vi "MinimalLiveExample.vi"() -> ()   [LabVIEW 2020]
uses:
  C:/Users/Public/Documents/Photometrics/TPM-LabVIEWSamples/Examples/2020/Dependencies/PVCamNET.dll
  Public/Documents/Photometrics/TPM-LabVIEWSamples/Examples/2020/Dependencies/PVCamNET.dll
panel:
  in  "Stop":bool
  out "Image Data":u16[][](array[numeric])
  out "Error":errorcluster
  out "Current Frame":u32
  out "Sensor Width":u32
  out "Sensor Height":u32
  out "Camera Name":string
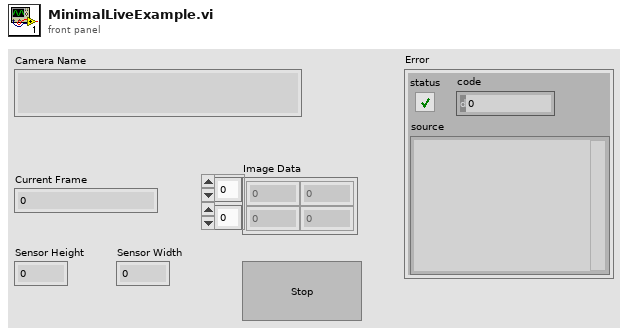
[diagram p1: front panel]
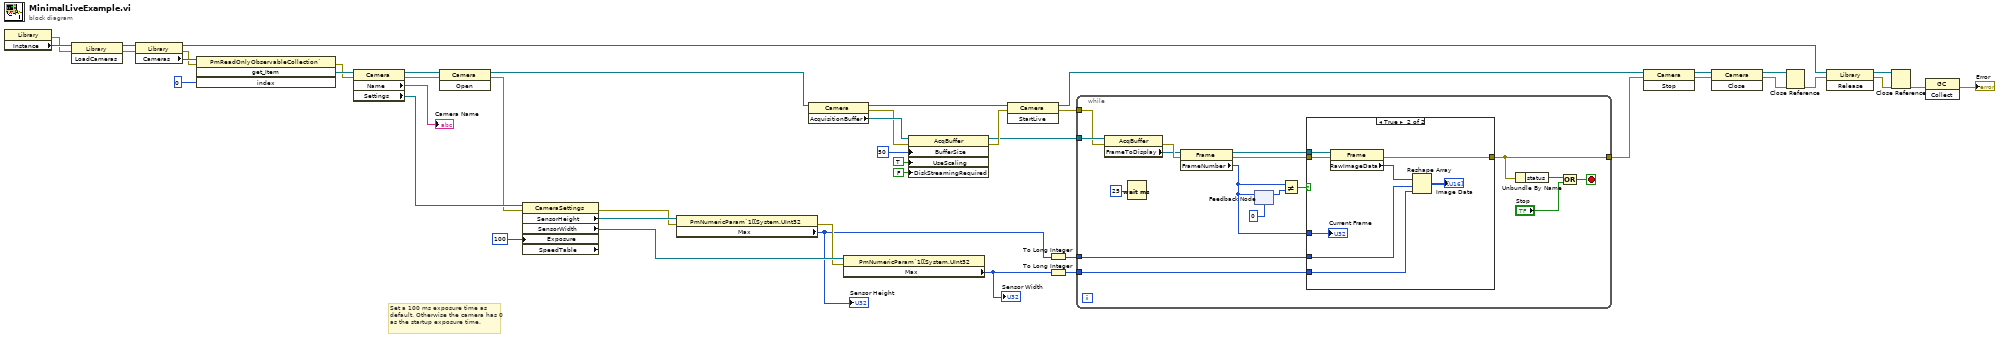
[diagram p0: block diagram]
diagram:
  # "Set a 100 ms exposure time as default. Otherwise the camera has 0 as the startup exposure time."
  n1 = property class="Library"() -> (error out=w42:errorcluster, "Instance"=w45:refnum<k24>)  [unwired: 2 in, 1 out]
  n2 = invoke class="Library" method="LoadCameras"(reference=w45, error in=w42) -> (reference out=w44:refnum<k24>, error out=w41:errorcluster)  [unwired: 1 in, 1 out]
  n3 = property class="Library"(reference=w44, error in=w41) -> (reference out=w34:refnum<k24>, error out=w40:errorcluster, "Cameras"=w43:refnum<k24>)
  n4 = invoke class="PmReadOnlyObservableCollection`" method="get_Item"(reference=w43, error in=w40, "index"=0) -> (error out=w38:errorcluster, "get_Item"=w39:refnum<k24>)  [unwired: 1 in, 2 out]
  n5 = property class="Camera"(reference=w39, error in=w38) -> (reference out=w36:refnum<k24>, error out=w33:errorcluster, "Name"=→"Camera Name":string, "Settings"=w37:refnum<k24>)
  n6 = invoke class="Camera" method="Open"(reference=w36, error in=w33) -> (reference out=w7:refnum<k24>, error out=w32:errorcluster)  [unwired: 1 in, 1 out]
  n7 = property class="CameraSettings" props=["SensorHeight", "SensorWidth", "Exposure", "SpeedTable"](reference=w37, error in=w32, "Exposure"=u32 100) -> (error out=w29:errorcluster, "SensorHeight"=w31:refnum<k24>, "SensorWidth"=w30:refnum<k24>)  [unwired: 2 out]
  n8 = property class="PmNumericParam`1[[System.UInt32"(reference=w31, error in=w29) -> (error out=w28:errorcluster, "Max"=w10:u32)  [unwired: 1 out]
  "Sensor Height" <- w10
  n9 = property class="Camera"(reference=w7) -> (reference out=w16:refnum<k24>, error out=w18:errorcluster, "AcquisitionBuffer"=w19:refnum<k24>)  [unwired: 1 in]
  n10 = property class="PmNumericParam`1[[System.UInt32"(reference=w30, error in=w28) -> ("Max"=w11:u32)  [unwired: 2 out]
  "Sensor Width" <- w11
  n11 = property class="AcqBuffer"(reference=w19, error in=w18, "BufferSize"=u32 50, "UseScaling"=TRUE, "DiskStreamingRequired"=FALSE) -> (reference out=w14:refnum<k24>, error out=w15:errorcluster)
  n12 = invoke class="Camera" method="StartLive"(reference=w16, error in=w15) -> (reference out=w2:refnum<k24>, error out=w13:errorcluster)  [unwired: 1 in, 1 out]
  n13 = To Long Integer(number=w10) -> (32bit integer=w9:i32)
  n14 = To Long Integer(number=w11) -> (32bit integer=w8:i32)
  n15 = while {
    tunnel: w14 -> [w60]
    tunnel: w13 -> [w59]
    tunnel: [w47] -> w4
    tunnel: w8 -> [w50]
    tunnel: w9 -> [w51]
    stop <- w57 stop-if-true
    n16 = property class="AcqBuffer"(reference=w60, error in=w59) -> (error out=w62:errorcluster, "FrameToDisplay"=w61:refnum<k24>)  [unwired: 1 out]
    n17 = Wait (ms)(milliseconds to wait=u32 25) -> ()  [unwired: 1 out]
    n18 = property class="Frame"(reference=w61, error in=w62) -> (reference out=w52:refnum<k24>, error out=w49:errorcluster, "FrameNumber"=w48:u32)
    n19 = feedback #1(u32 0 ("FrameNumber")) -> (w54:u32)
    n20 = feedback-in #1(w48) -> ()
    n21 = Not Equal?(x=w48, y=w54) -> (x != y?=w53:bool)
    n22 = case shown="True" w53 {
      tunnel: w52 -> [_ w71]
      tunnel: w51 -> [_ w70]
      tunnel: w50 -> [_ w69]
      tunnel: w49 -> [w63 w68]
      tunnel: [w63 w66] -> w47
      tunnel: w48 -> [_ w67]
      frame False {
      }
      frame True {
        n23 = property class="Frame"(reference=w71, error in=w68) -> (error out=w66:errorcluster, "RawImageData"=w64:u16[])  [unwired: 1 out]
        n24 = Reshape Array(w64, w70, w69) -> (→"Image Data":u16[][])
        "Current Frame" <- w67
      }
    }
    n25 = Unbundle By Name(w47) -> ("status"=w58:bool)
    n26 = Or(x=w58, y="Stop") -> (x .or. y?=w57:bool)
  }
  n27 = invoke class="Camera" method="Stop"(reference=w2, error in=w4) -> (reference out=w3:refnum<k24>, error out=w1:errorcluster)  [unwired: 1 in, 1 out]
  n28 = invoke class="Camera" method="Close"(reference=w3, error in=w1) -> (reference out=w24:refnum<k24>, error out=w22:errorcluster)  [unwired: 1 in, 1 out]
  n29 = Close Reference(reference=w24, error in (no error)=w22) -> (error out=w21:errorcluster)
  n30 = invoke class="Library" method="Release"(reference=w34, error in=w21) -> (reference out=w23:refnum<k24>, error out=w26:errorcluster)  [unwired: 1 in, 1 out]
  n31 = Close Reference(reference=w23, error in (no error)=w26) -> (error out=w25:errorcluster)
  n32 = invoke class="GC" method="Collect"(error in=w25) -> (error out=→"Error":errorcluster)  [unwired: 2 in, 2 out]
